vi "OP_PW.vi"(2 "error in":errorcluster, 3 "Op_name":string, 4 "Path":path) -> (0 "error out":errorcluster, 1 "Password":string)   [LabVIEW 2024]
uses:
  Launcher_DTU.lvlib
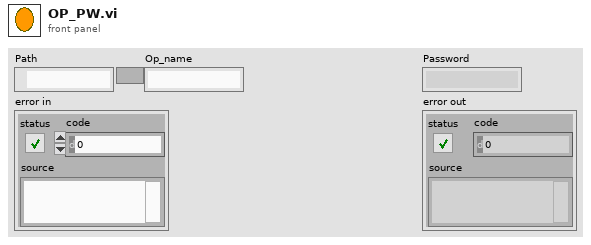
[diagram p1: front panel]
types:
  T1 = cluster{"Operator name":string, "Password":string}[]
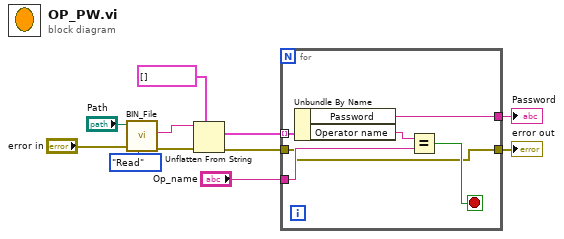
[diagram p0: block diagram]
diagram:
  n1 = call "BIN_File.vi"("Enum"=enum16{"Read", "Write"}."Read", "error in"="error in", "Path"="Path") -> ("error out"=w8:errorcluster, "data out"=w7:string)  [unwired: 7 in]
  n2 = Unflatten From String(type=T1 [], binary string=w7, error in (no error)=w8) -> (value=w5:T1, error out=w4:errorcluster)  [unwired: 2 in, 1 out]
  n3 = for {
    tunnel: w5 -> [w17] mode=indexing
    tunnel: w4 -> [w12]
    tunnel: "Op_name" -> [w15]
    tunnel: [w13] -> w2
    tunnel: [w12] -> w1
    stop <- w14 stop-if-true
    n4 = Unbundle By Name(w17) -> ("Password"=w13:string, "Operator name"=w16:string)
    n5 = Equal?(x=w16, y=w15) -> (x = y?=w14:bool)
  }
  "Password" <- w2
  "error out" <- w1
